vi "Resize Panel to Pane.vi"(8 "error in (no error)":errorcluster, 10 "Apply Recursively? (F)":bool, 11 "RandomDataChart In":refnum<class "BasicChartBinding.lvclass">) -> (0 "error out":errorcluster, 3 "RandomDataChart Out":refnum<class "BasicChartBinding.lvclass">)   [LabVIEW 2018, in "TestViewables.lvlib" / "BasicChartBinding.lvclass"]
doc: "<License>\nCopyright © 2017 Composed Systems, LLC | All rights reserved\nwww.composed.io\n\nAuthor: Ethan Stern <ethan.stern@composed.io>\n\nThis software is provided \"AS IS\" WITHOUT WARRANTIES, either express or implied, AND IS FOR EDUCATIONAL PURPOSES ONLY.\n</License>"
uses:
  BasicChartBinding.lvclass
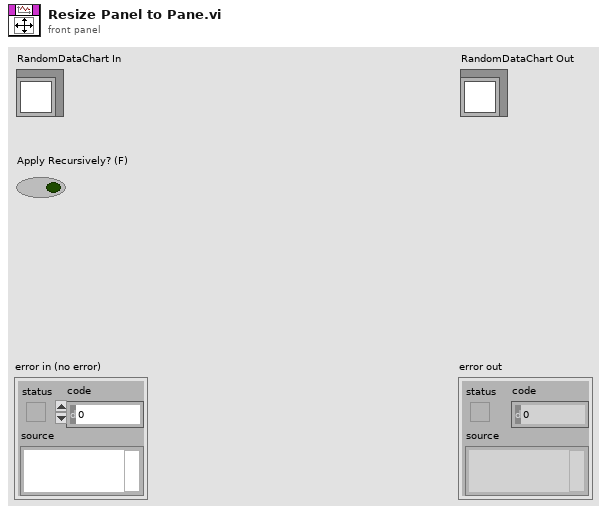
[diagram p1: front panel]
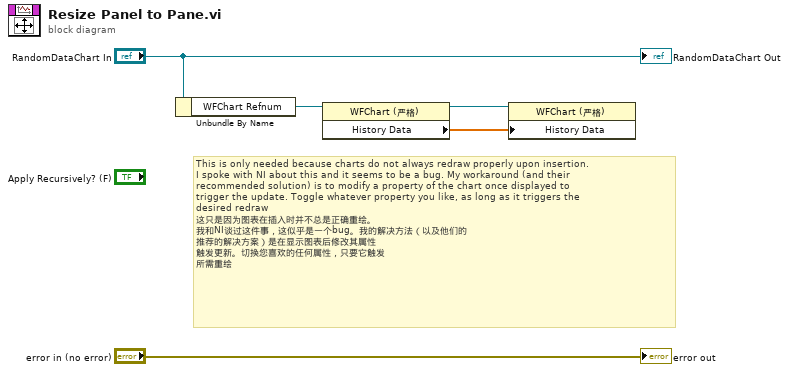
[diagram p0: block diagram]
diagram:
  # "This is only needed because charts do not always redraw properly upon insertion.\nI spoke with NI about this and it seems to be a bug. My workaround (and their\nrecommended solution) is to modify a property of the chart once displayed to\ntrigger the update. Toggle whatever property you like, as long as it triggers the\ndesired redraw\n这只是因为图表在插入时并不总是正确重绘。\n我和NI谈过这件事，这似乎是一个bug。我的解决方法（以及他们的\n推荐的解决方案）是在显示图表后修改其属性\n触发更新。切换您喜欢的任何属性，只要它触发\n所需重绘"
  n1 = Unbundle By Name("RandomDataChart In") -> ("WFChart Refnum"=w3:refnum<vi>)
  n2 = property class="WFChart (严格)"(reference=w3) -> (reference out=w2:refnum<vi>, "History Data"=w1:dbl[])  [unwired: 1 in, 1 out]
  n3 = property class="WFChart (严格)"(reference=w2, "History Data"=w1) -> ()  [unwired: 1 in, 2 out]
  "error out" <- "error in (no error)"
  "RandomDataChart Out" <- "RandomDataChart In"
